vi "Edit VI Constants.vi"(8 "error in":errorcluster, 10 "relative path of VI to edit":path, 11 "custom device path":path) -> (0 "error out":errorcluster, 3 "custom device path out":path)   [LabVIEW 2020, in "Template Tool.lvlib"]
uses:
  Template Tool.lvlib
  Template Tool Global.vi
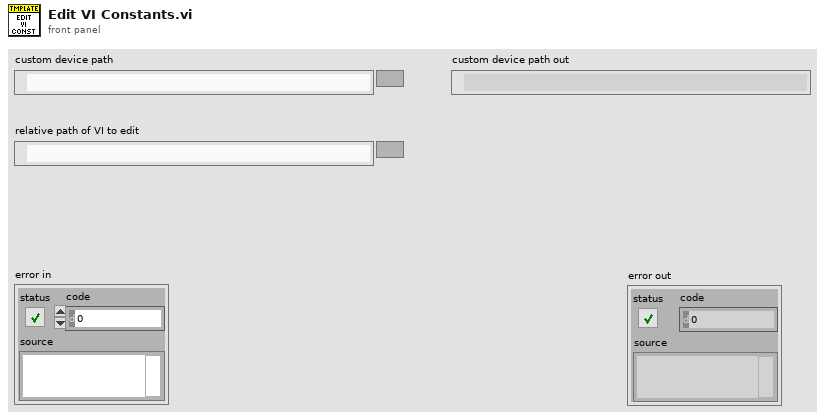
[diagram p1: front panel]
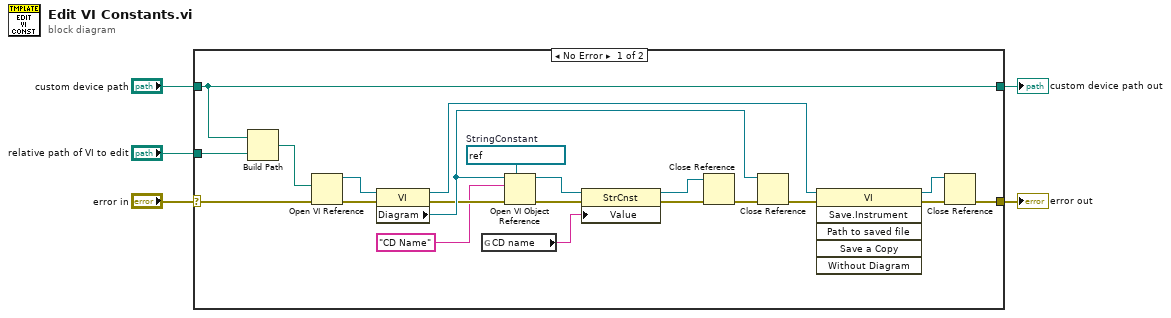
[diagram p0: block diagram]
diagram:
  n1 = case shown="No Error" "error in" {
    selector: "error in" -> [w20 w27]
    tunnel: [w13 w27] -> w5
    tunnel: "custom device path" -> [w21 w28]
    tunnel: "relative path of VI to edit" -> [w22 _]
    tunnel: [w21 w28] -> w2
    frame No Error {
      w10 = refnum<vi> refnum  # StringConstant
      n2 = Build Path(base path=w21, name or relative path=w22) -> (appended path=w24:path)
      n3 = Open VI Reference(vi path=w24, error in (no error)=w20) -> (vi reference=w25:refnum<vi>, error out=w26:errorcluster)  [unwired: 4 in]
      n4 = property class="VI"(reference=w25, error in=w26) -> (reference out=w23:refnum<vi>, error out=w12:errorcluster, "Diagram"=w18:refnum<vi>)
      n5 = global read "Template Tool Global.vi" "CD name"() -> (w6:string)
      n6 = Open VI Object Reference(7:w10, 8:w12, 10:"CD Name" ("Class Name"), 11:w18) -> (0:w9:errorcluster, 3:w8:refnum<vi>)
      n7 = property class="StrCnst"(reference=w8, error in=w9, "Value"=w6) -> (reference out=w7:refnum<vi>, error out=w17:errorcluster)
      n8 = Close Reference(reference=w7, error in (no error)=w17) -> (error out=w19:errorcluster)
      n9 = Close Reference(reference=w18, error in (no error)=w19) -> (error out=w16:errorcluster)
      n10 = invoke class="VI" method="Save.Instrument"(reference=w23, error in=w16) -> (reference out=w15:refnum<vi>, error out=w14:errorcluster)  [unwired: 4 in, 4 out]
      n11 = Close Reference(reference=w15, error in (no error)=w14) -> (error out=w13:errorcluster)
    }
    frame Error {
    }
  }
  "error out" <- w5
  "custom device path out" <- w2
